vi "createCommands.vi"(8 "error in (no error)":errorcluster, 11 "SAL_Events in":refnum<class "SAL_Events.lvclass">) -> (0 "error out":errorcluster, 3 "SAL_Events out":refnum<class "SAL_Events.lvclass">)   [LabVIEW 2015, in "SAL_Events.lvclass"]
uses:
  SAL_Events.lvclass
  typedefs/commandsEvents.ctl
  SALLV_dome/DataTypes/command_start.ctl
  SALLV_dome/DataTypes/command_disable.ctl
  SALLV_dome/DataTypes/command_enable.ctl
  SALLV_dome/DataTypes/command_exitControl.ctl
  SALLV_dome/DataTypes/command_standby.ctl
  SALLV_dome/DataTypes/command_stop.ctl
  SALLV_dome/DataTypes/command_Move.ctl
  SALLV_dome/DataTypes/command_Crawl.ctl
  SALLV_dome/DataTypes/command_SetLouvers.ctl
  SALLV_dome/DataTypes/command_Park.ctl
  SALLV_dome/DataTypes/command_StopShutter.ctl
  SALLV_dome/DataTypes/command_OpenShutter.ctl
  SALLV_dome/DataTypes/command_CloseShutter.ctl
  SAL_Events.lvclass/SAL_Events.ctl
  SALLV_dome/SALLV_dome.lvlib
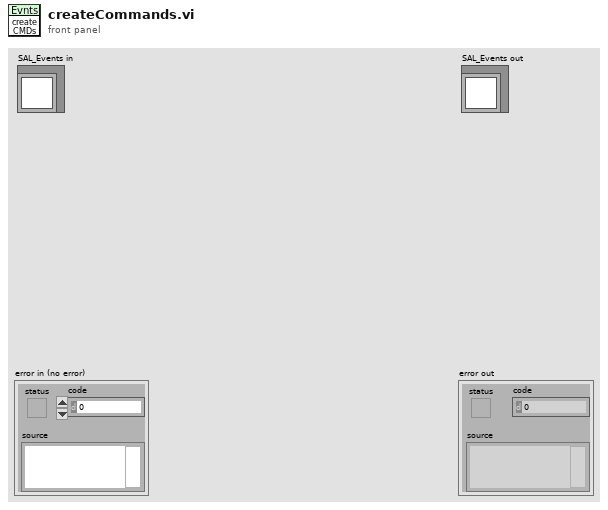
[diagram p1: front panel]
types:
  T1 = typedef "SALLV_dome.lvlib/command_CloseShutter.ctl" = cluster{"state":bool}
  T2 = typedef "SALLV_dome.lvlib/command_OpenShutter.ctl" = cluster{"state":bool}
  T3 = typedef "SALLV_dome.lvlib/command_StopShutter.ctl" = cluster{"state":bool}
  T4 = typedef "SALLV_dome.lvlib/command_Park.ctl" = cluster{"state":bool}
  T5 = typedef "SALLV_dome.lvlib/command_SetLouvers.ctl" = cluster{"position[34]":i32[]}
  T6 = typedef "SALLV_dome.lvlib/command_Crawl.ctl" = cluster{"azPosition":dbl, "elPosition":dbl, "demandTime":i32}
  T7 = typedef "SALLV_dome.lvlib/command_Move.ctl" = cluster{"azimuth":dbl, "elevation":dbl}
  T8 = typedef "SALLV_dome.lvlib/command_stop.ctl" = cluster{"state":bool}
  T9 = typedef "SALLV_dome.lvlib/command_standby.ctl" = cluster{"state":bool}
  T10 = typedef "SALLV_dome.lvlib/command_exitControl.ctl" = cluster{"state":bool}
  T11 = typedef "SALLV_dome.lvlib/command_enable.ctl" = cluster{"state":bool}
  T12 = typedef "SALLV_dome.lvlib/command_disable.ctl" = cluster{"state":bool}
  T13 = typedef "SALLV_dome.lvlib/command_start.ctl" = cluster{"configuration":string}
  T14 = typedef "commandsEvents.ctl" = cluster{"start":refnum<user-event>, "disable":refnum<user-event>, "enable":refnum<user-event>, "exitControl":refnum<user-event>, "standby":refnum<user-event>, "stop":refnum<user-event>, "move":refnum<user-event>, "crawl":refnum<user-event>, "setLouvers":refnum<user-event>, "Park":refnum<user-event>, "StopShutter":refnum<user-event>, "OpenShutter":refnum<user-event>, "CloseShutter":refnum<user-event>}
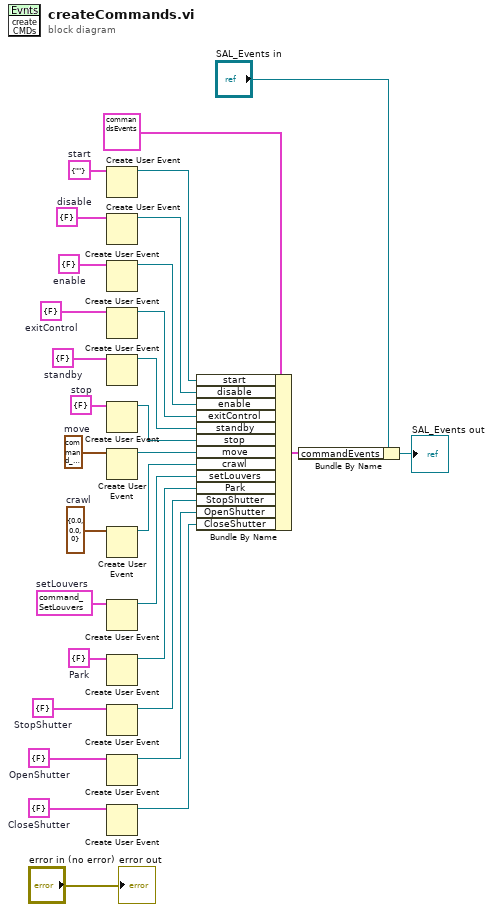
[diagram p0: block diagram]
diagram:
  w5 = T1 {"state"=FALSE}  # CloseShutter
  w6 = T2 {"state"=FALSE}  # OpenShutter
  w7 = T3 {"state"=FALSE}  # StopShutter
  w8 = T4 {"state"=FALSE}  # Park
  w9 = T5 {"position[34]"=[0, 0, 0, 0, 0, 0, 0, 0, 0, 0, 0, 0, 0, 0, 0, 0, 0, 0, 0, 0, 0, 0, 0, 0, 0, 0, 0, 0, 0, 0, 0, 0, 0, 0]}  # setLouvers
  w10 = T6 {"azPosition"=0.0, "elPosition"=0.0, "demandTime"=0}  # crawl
  w11 = T7 {"azimuth"=0.0, "elevation"=0.0}  # move
  w12 = T8 {"state"=FALSE}  # stop
  w13 = T9 {"state"=FALSE}  # standby
  w14 = T10 {"state"=FALSE}  # exitControl
  w15 = T11 {"state"=FALSE}  # enable
  w16 = T12 {"state"=FALSE}  # disable
  w17 = T13 {"configuration"=""}  # start
  n1 = Create User Event(user event datatype=w17) -> (user event=w29:refnum<user-event>)  [unwired: 1 in, 1 out]
  n2 = Create User Event(user event datatype=w16) -> (user event=w28:refnum<user-event>)  [unwired: 1 in, 1 out]
  n3 = Create User Event(user event datatype=w15) -> (user event=w27:refnum<user-event>)  [unwired: 1 in, 1 out]
  n4 = Create User Event(user event datatype=w14) -> (user event=w26:refnum<user-event>)  [unwired: 1 in, 1 out]
  n5 = Create User Event(user event datatype=w13) -> (user event=w25:refnum<user-event>)  [unwired: 1 in, 1 out]
  n6 = Create User Event(user event datatype=w12) -> (user event=w24:refnum<user-event>)  [unwired: 1 in, 1 out]
  n7 = Create User Event(user event datatype=w11) -> (user event=w23:refnum<user-event>)  [unwired: 1 in, 1 out]
  n8 = Create User Event(user event datatype=w10) -> (user event=w22:refnum<user-event>)  [unwired: 1 in, 1 out]
  n9 = Create User Event(user event datatype=w9) -> (user event=w21:refnum<user-event>)  [unwired: 1 in, 1 out]
  n10 = Create User Event(user event datatype=w8) -> (user event=w4:refnum<user-event>)  [unwired: 1 in, 1 out]
  n11 = Create User Event(user event datatype=w7) -> (user event=w3:refnum<user-event>)  [unwired: 1 in, 1 out]
  n12 = Create User Event(user event datatype=w6) -> (user event=w2:refnum<user-event>)  [unwired: 1 in, 1 out]
  n13 = Create User Event(user event datatype=w5) -> (user event=w1:refnum<user-event>)  [unwired: 1 in, 1 out]
  n14 = Bundle By Name(cluster=T14 {"start"=refnum, "disable"=refnum, "enable"=refnum, "exitControl"=refnum, "standby"=refnum, "stop"=refnum, "move"=refnum, "crawl"=refnum, "setLouvers"=refnum, "Park"=refnum, "StopShutter"=refnum, "OpenShutter"=refnum, "CloseShutter"=refnum} ("commandEvents"), "start"=w29, "disable"=w28, "enable"=w27, "exitControl"=w26, "standby"=w25, "stop"=w24, "move"=w23, "crawl"=w22, "setLouvers"=w21, "Park"=w4, "StopShutter"=w3, "OpenShutter"=w2, "CloseShutter"=w1) -> (w18:T14)
  n15 = Bundle By Name(cluster="SAL_Events in", "commandEvents"=w18) -> (→"SAL_Events out":refnum<class "SAL_Events.lvclass">)
  "error out" <- "error in (no error)"
